vi "Software Update HCC Build The Latest Path.vi"(8 "Error In":errorcluster, 10 "Path Build List Sub Input":path, 11 "Latest Exe Files":path) -> (0 "Error Out":errorcluster, 3 "Updated Path":path)   [LabVIEW 2016]
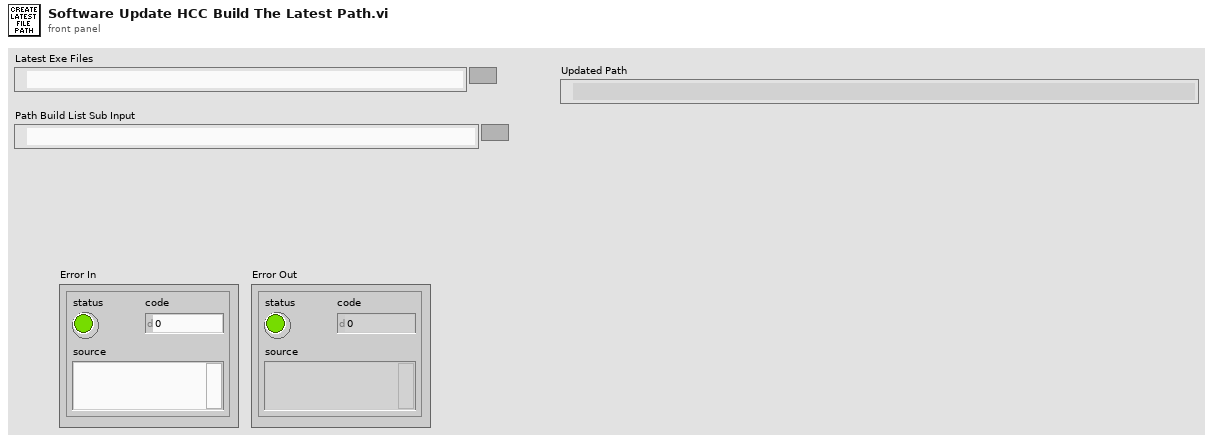
[diagram p1: front panel]
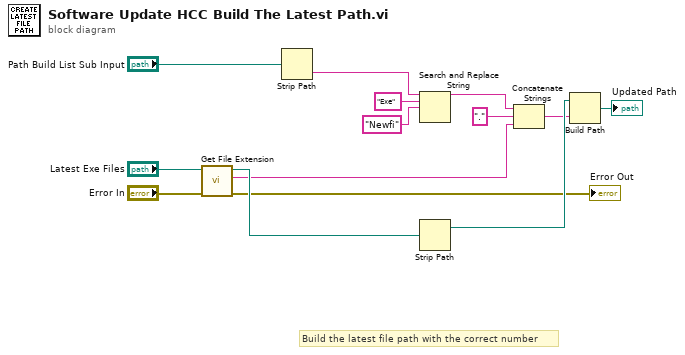
[diagram p0: block diagram]
diagram:
  # "Build the latest file path with the correct number"
  n1 = call <vilib>:"Get File Extension.vi"("error in (no error)"="Error In", "file"="Latest Exe Files") -> ("error out"=→"Error Out":errorcluster, "lowercase file extension"=w8:string, "dup file"=w12:path)  [unwired: 5 in, 2 out]
  n2 = Strip Path(path="Path Build List Sub Input") -> (name=w4:string)  [unwired: 1 out]
  n3 = Search and Replace String(input string=w4, search string="Exe", replace string="Newfi" ("regular expression")) -> (result string=w14:string)  [unwired: 5 in, 3 out]
  n4 = Strip Path(path=w12) -> (stripped path=w13:path)  [unwired: 1 out]
  n5 = Concatenate Strings(w14, "." ("string"), w8) -> (w10:string)
  n6 = Build Path(base path=w13, name or relative path=w10) -> (appended path=→"Updated Path":path)
